vi "Module Name--constant.vi"() -> (3 "Module Name":string)   [LabVIEW 2023, in "DAQ.lvlib"]
doc: "Return the name of the module that owns this VI. \n_____\nBased on DQMH Project Template 6.1.0.94."
uses:
  DAQ.lvlib
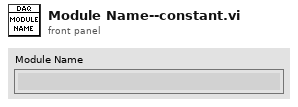
[diagram p1: front panel]
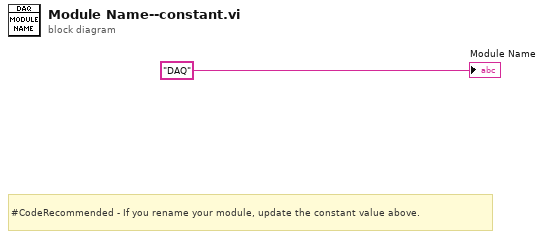
[diagram p0: block diagram]
diagram:
  # "#CodeRecommended - If you rename your module, update the constant value above."
  "Module Name" <- "DAQ"
